vi "New JSON Web Token.vi"(8 "error in (no error)":errorcluster, 9 "Issuer URI path (component)":string, 10 "Base64url JWT string":string, 11 "Client ID":string) -> (0 "error out":errorcluster, 1 "Valid JWT?":bool, 2 "registered claims":T2, 3 "JSONWebToken out":refnum<class "JSONWebToken.lvclass">, 4 "date/time claims":T1, 5 "JWT Claims (JSON)":string)   [LabVIEW 2017, in "JSONWebToken.lvclass"]
doc: "Validates a Base64URL encoded JWT string and returns a deserialized LabVIEW object."
uses:
  JSONWebToken.lvclass
  JWT registered Claims -- cluster.ctl
  JWT standard OpenID Claims -- ring.ctl
  JSONWebToken.lvclass/JSONWebToken.ctl
  Parse ID Token elements.vi
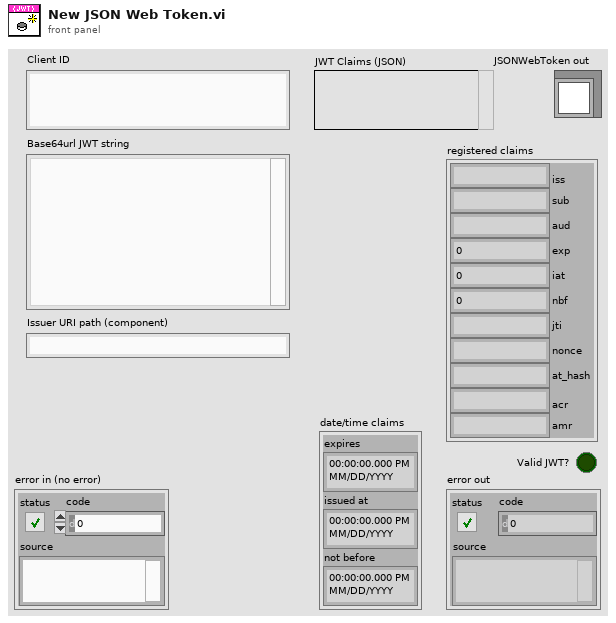
[diagram p1: front panel]
types:
  T1 = cluster{"expires":timestamp, "issued at":timestamp, "not before":timestamp}
  T2 = typedef "JSONWebToken.lvclass/JWT registered Claims -- cluster.ctl" = cluster{"iss":string, "sub":string, "aud":string, "exp":i32, "iat":i32, "nbf":i32, "jti":string, "nonce":string, "at_hash":string, "acr":string, "amr":string}
  T3 = typedef "JSONWebToken.lvclass/JWT standard OpenID Claims -- ring.ctl" = string
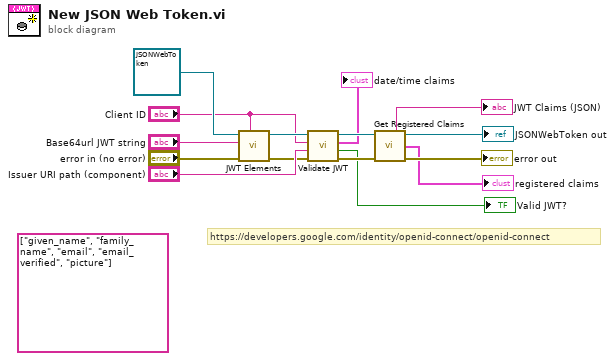
[diagram p0: block diagram]
diagram:
  (unwired) T3[] ["given_name", "family_name", "email", "email_verified", "picture"]
  # "https://developers.google.com/identity/openid-connect/openid-connect"
  n1 = call "JWT Elements.vi"("Client ID"="Client ID", "error in (no error)"="error in (no error)", "id_token"="Base64url JWT string", "JSONWebToken in"=refnum<class "JSONWebToken.lvclass"> refnum ("JSONWebToken.lvclass")) -> ("error out"=w10:errorcluster, "JSONWebToken out"=w11:refnum<class "JSONWebToken.lvclass">)  [unwired: 6 in]
  n2 = call "Validate JWT.vi"("error in (no error)"=w10, "Issuer URI path (component)"="Issuer URI path (component)", "Client ID"="Client ID", "JSONWebToken in"=w11) -> ("error out"=w7:errorcluster, "Valid JWT?"=→"Valid JWT?":bool, "date/time claims"=→"date/time claims":T1, "JSONWebToken out"=w8:refnum<class "JSONWebToken.lvclass">)  [unwired: 4 in]
  n3 = call "Get Registered Claims.vi"("JSONWebToken in"=w8, "error in (no error)"=w7) -> ("payload (JSON)"=→"JWT Claims (JSON)":string, "JSONWebToken out"=→"JSONWebToken out":refnum<class "JSONWebToken.lvclass">, "registered claims"=→"registered claims":T2, "error out"=→"error out":errorcluster)  [unwired: 10 in]
